vi "Primary Flow Characteristics.vi"(0 "Primary Cold Density":dbl, 1 "Core Channel Equivalent Diameter":dbl, 2 "Downcomer Gap":dbl, 3 "Velocity (m/s) in":dbl, 4 "Velocity (m/s) 4":dbl, 5 "Velocity (m/s) 3":dbl, 6 "Velocity":dbl, 8 "Primary Hot Density":dbl, 9 "FLiBe Viscosity (Pa-s) 3":dbl, 10 "Primary Average Density":dbl, 11 "FLiBe Viscosity (Pa-s) in":dbl, 12 "MHX Tube Diameter":dbl, 13 "FLiBe Viscosity":dbl, 14 "Pipe Diameter":dbl) -> (16 "AC Reynolds Number":dbl, 18 "CD Reynolds Number":dbl, 19 "GA Reynolds Number":dbl, 20 "AC Friction Factor":dbl, 21 "DF Reynolds Number":dbl, 22 "CD Friction Factor":dbl, 23 "FG Reynolds Number":dbl, 24 "DF Friction Factor":dbl, 25 "FG Friction Factor":dbl, 26 "GA Friction Factor":dbl)   [LabVIEW 2019]
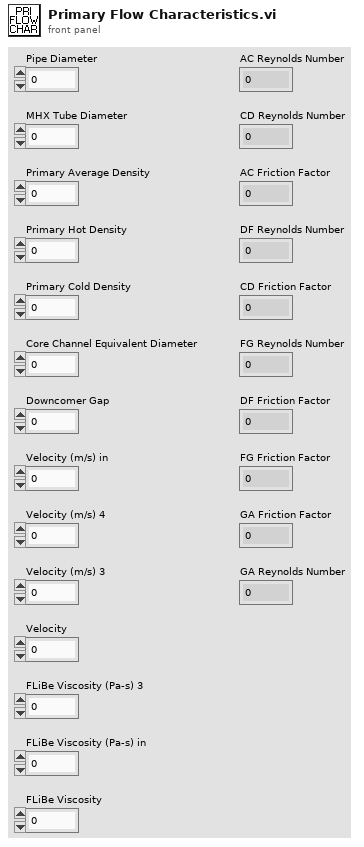
[diagram p1: front panel]
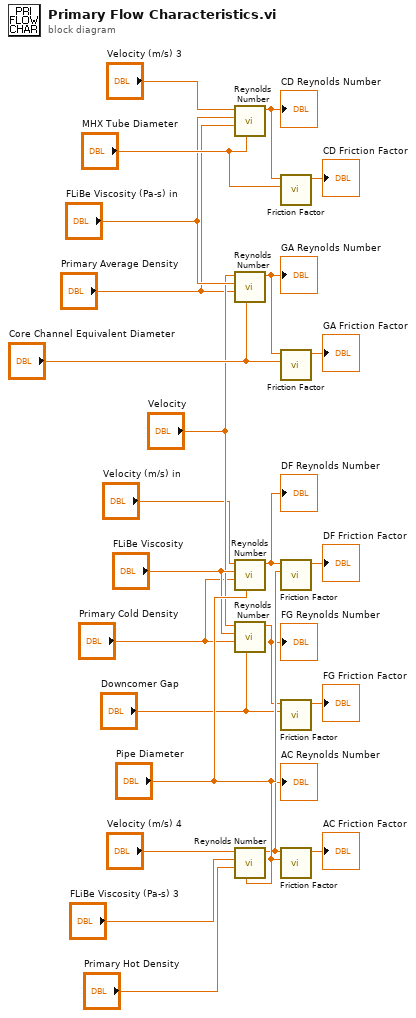
[diagram p0: block diagram]
diagram:
  n1 = call "Reynolds Number.vi"("Effective Length (m)"="MHX Tube Diameter", "Density (kg/m^3)"="Primary Average Density", "Viscosity (Pa-s)"="FLiBe Viscosity (Pa-s) in", "Velocity (m/s)"="Velocity (m/s) 3") -> ("Reynolds Number"=w14:dbl)  [unwired: 7 in]
  "CD Reynolds Number" <- w14
  n2 = call "Reynolds Number.vi"("Effective Length (m)"="Core Channel Equivalent Diameter", "Density (kg/m^3)"="Primary Average Density", "Viscosity (Pa-s)"="FLiBe Viscosity (Pa-s) in", "Velocity (m/s)"="Velocity") -> ("Reynolds Number"=w20:dbl)  [unwired: 7 in]
  "GA Reynolds Number" <- w20
  n3 = call "Reynolds Number.vi"("Effective Length (m)"="Pipe Diameter", "Density (kg/m^3)"="Primary Cold Density", "Viscosity (Pa-s)"="FLiBe Viscosity", "Velocity (m/s)"="Velocity (m/s) in") -> ("Reynolds Number"=w18:dbl)  [unwired: 7 in]
  "DF Reynolds Number" <- w18
  n4 = call "Reynolds Number.vi"("Effective Length (m)"="Downcomer Gap", "Density (kg/m^3)"="Primary Cold Density", "Viscosity (Pa-s)"="FLiBe Viscosity", "Velocity (m/s)"="Velocity") -> ("Reynolds Number"=w19:dbl)  [unwired: 7 in]
  "FG Reynolds Number" <- w19
  n5 = call "Reynolds Number.vi"("Effective Length (m)"="Pipe Diameter", "Density (kg/m^3)"="Primary Hot Density", "Viscosity (Pa-s)"="FLiBe Viscosity (Pa-s) 3", "Velocity (m/s)"="Velocity (m/s) 4") -> ("Reynolds Number"=w11:dbl)  [unwired: 7 in]
  "AC Reynolds Number" <- w11
  n6 = call "Friction Factor.vi"("Effective Length"="MHX Tube Diameter", "Reynolds Number"=w14) -> ("Friction Factor"=→"CD Friction Factor":dbl)  [unwired: 9 in]
  n7 = call "Friction Factor.vi"("Effective Length"="Core Channel Equivalent Diameter", "Reynolds Number"=w20) -> ("Friction Factor"=→"GA Friction Factor":dbl)  [unwired: 9 in]
  n8 = call "Friction Factor.vi"("Effective Length"="Pipe Diameter", "Reynolds Number"=w18) -> ("Friction Factor"=→"DF Friction Factor":dbl)  [unwired: 9 in]
  n9 = call "Friction Factor.vi"("Effective Length"="Downcomer Gap", "Reynolds Number"=w19) -> ("Friction Factor"=→"FG Friction Factor":dbl)  [unwired: 9 in]
  n10 = call "Friction Factor.vi"("Effective Length"="Pipe Diameter", "Reynolds Number"=w11) -> ("Friction Factor"=→"AC Friction Factor":dbl)  [unwired: 9 in]
